vi "Param_Stack.vi"() -> ()   [LabVIEW 2020]
panel:
  in  "NbPASS":string
  out "Ton":dbl
  out "Is3P4S?":bool
  out "testDCIR?":bool
  out "VmaxPostDcir":dbl
  out "VminPostDcir":dbl
  out "Current":dbl
  out "Vmaxintraplus":dbl
  out "Vminintraplus":dbl
  out "Vmaxintramoins":dbl
  out "Vminintramoins":dbl
  out "TempMinDcir":dbl
  out "TempMaxDcir":dbl
  out "Vmin dcir":dbl
  out "Vmax dcir":dbl
  out "DeltamV":dbl
  out "DeltaC":dbl
  out "DeltamVintra":dbl
  out "Rmax":dbl
  out "Rminmili":dbl
  out "Rmaxmili":dbl
  out "OCVVmin":dbl
  out "OCVVmax":dbl
  in  "QRROOT":string
  in  "RefFichierStack on utilise plusssssssssss":string
  # "Hioki BT3562"
  # "DCIR"
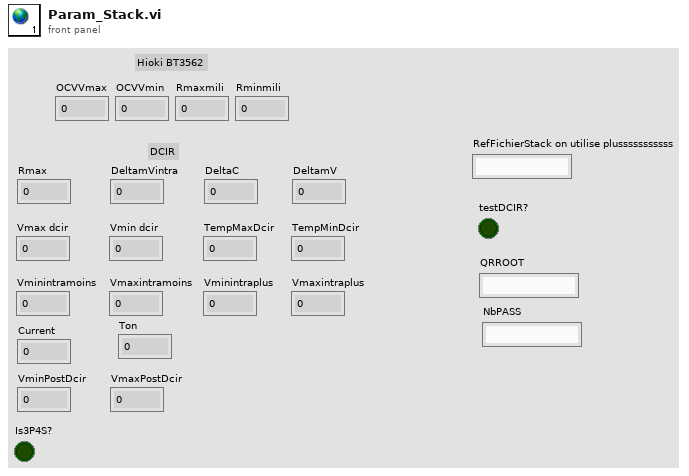
[diagram p1: front panel]
diagram:
